vi "MarcusAndMathiasMeetsGoogle.vi"(7 "language":enum16{"de", "en", "sk"}(ring)=enum."en", 8 "error in (no error)":errorcluster, 11 "Input Words":string[](array[string])) -> (0 "error out":errorcluster, 3 "result":string[](array[string]))   [LabVIEW 2015]
uses:
  <vilib>/httpClient/LabVIEWHTTPClient.lvlib
panel:
  in  "Test Value":bool
  out "Numeric":i32
  out "after substring 2":string
  out "json":string
  out "length":i32
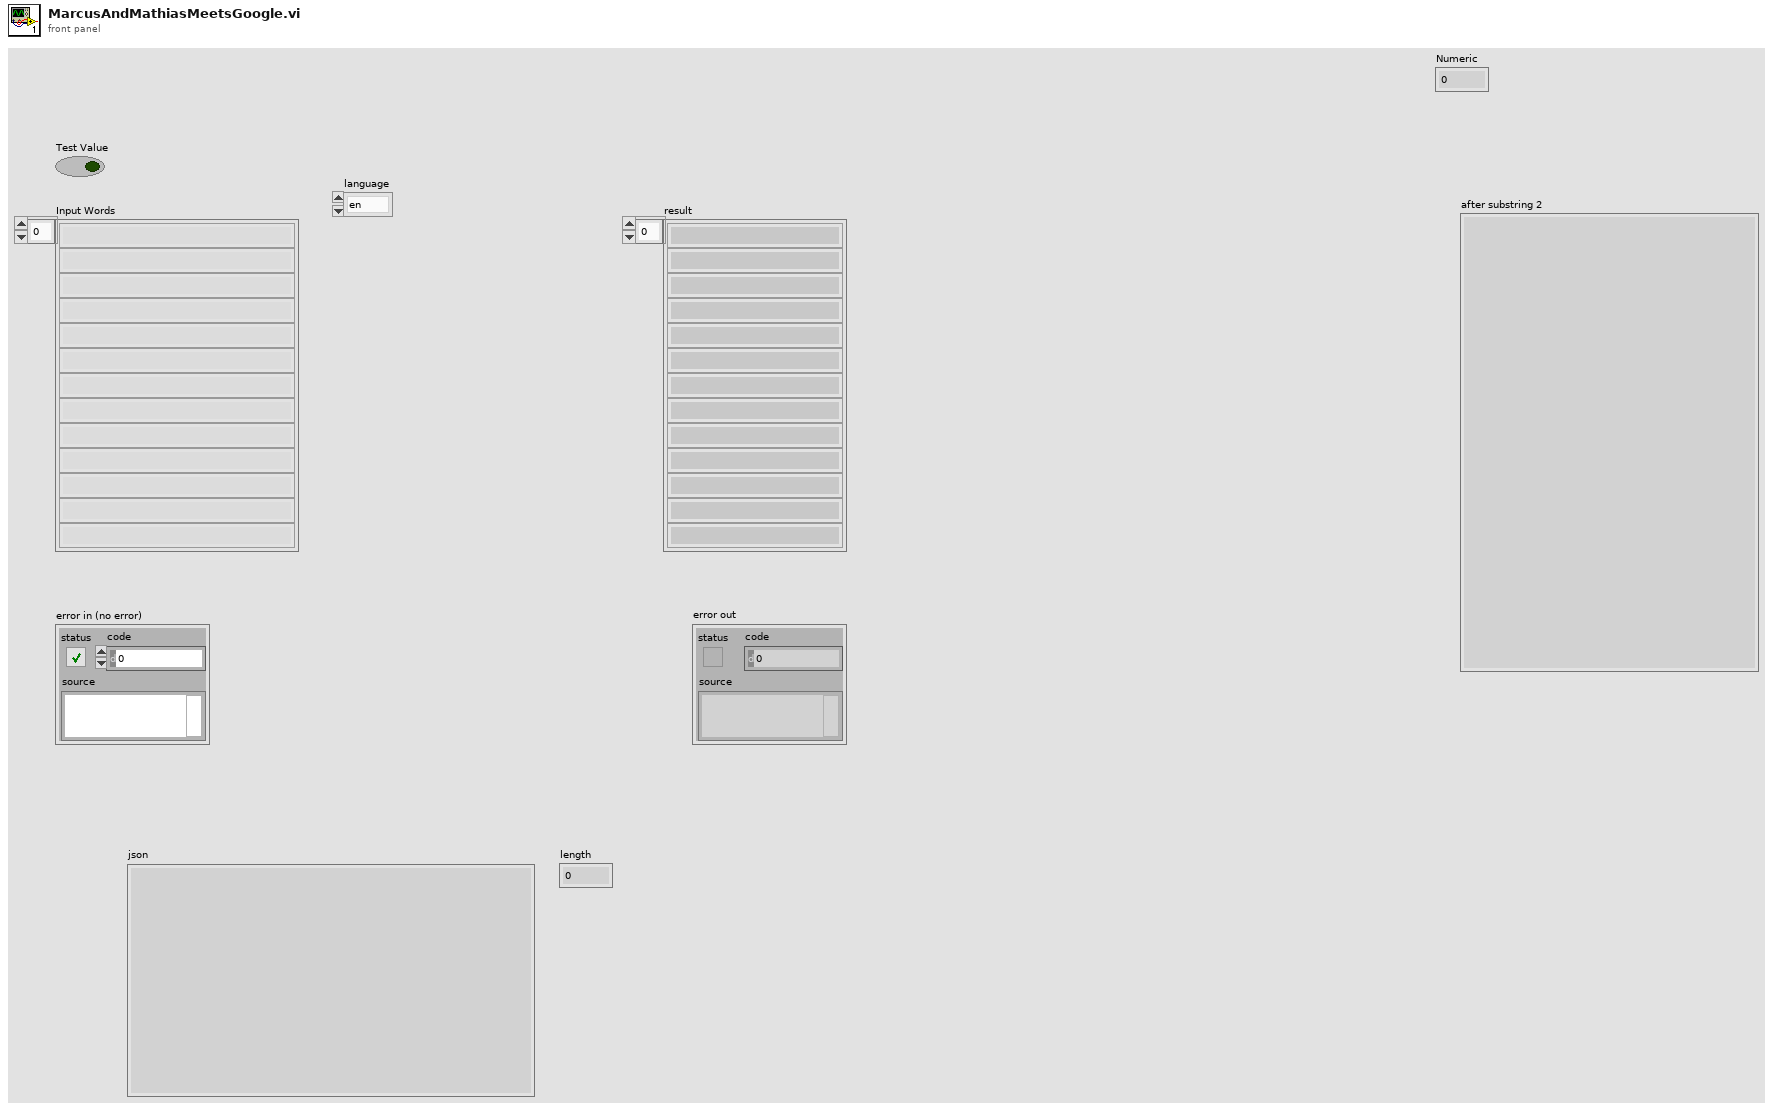
[diagram p1: front panel]
types:
  T1 = typedef "LabVIEWHTTPClient.lvlib/ClientHandle.ctl" = refnum<k1>
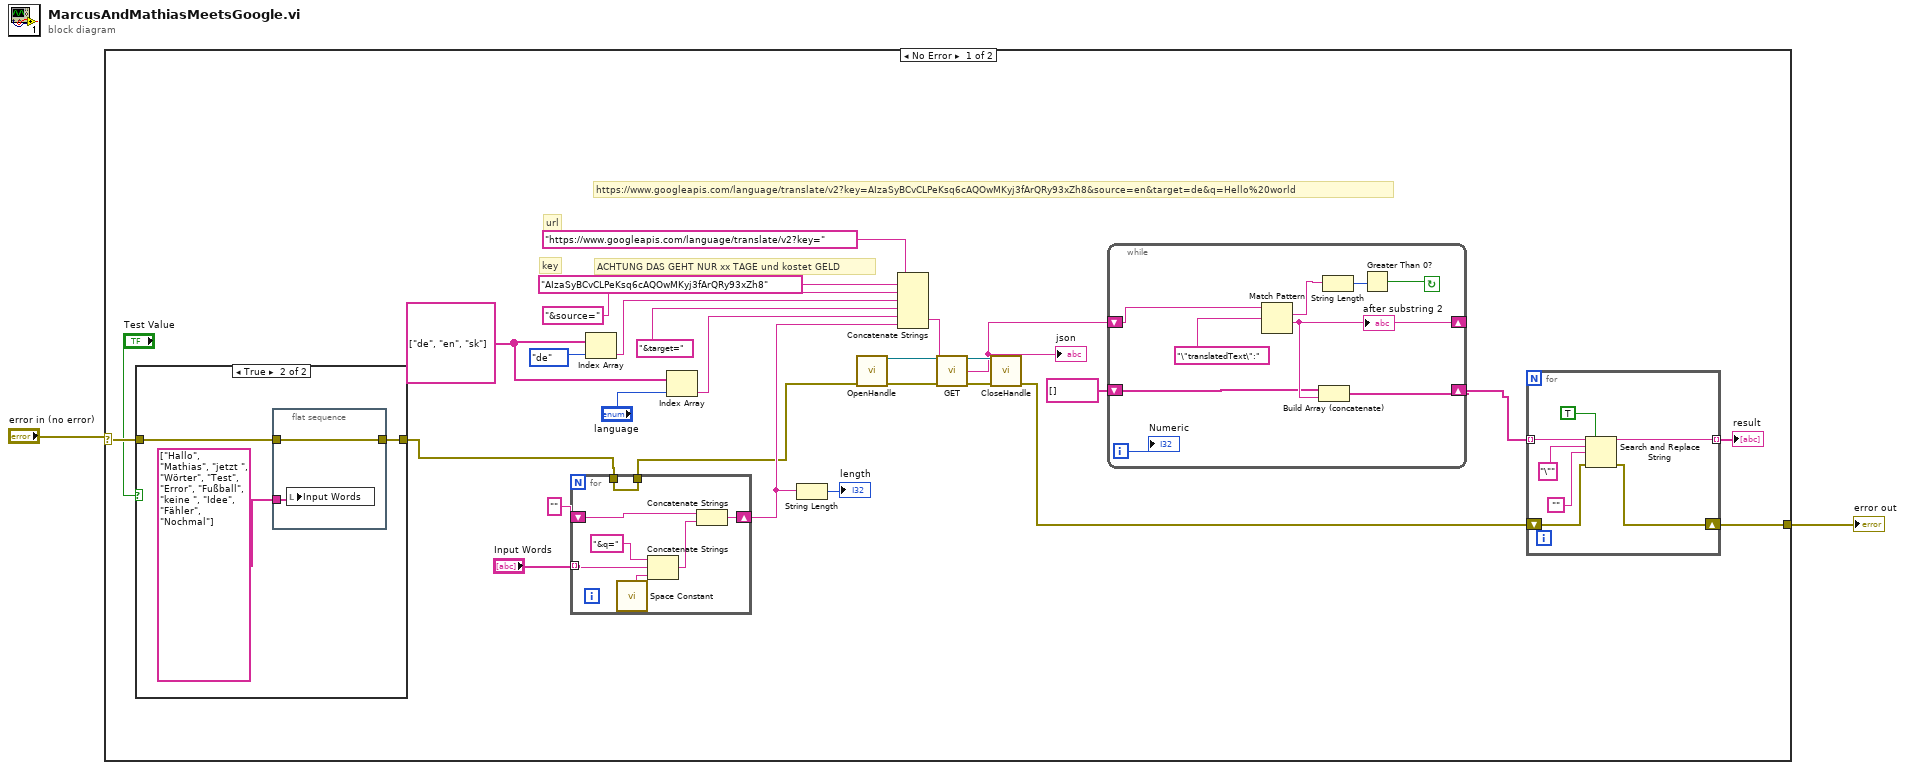
[diagram p0: block diagram]
diagram:
  n1 = case shown="No Error" "error in (no error)" {
    selector: "error in (no error)" -> [w8 w60]
    tunnel: [w7 w60] -> w1
    frame No Error {
      w19 = string[] ["de", "en", "sk"]
      # "ACHTUNG DAS GEHT NUR xx TAGE und kostet GELD"
      # "key"
      # "url"
      # "https://www.googleapis.com/language/translate/v2?key=AIzaSyBCvCLPeKsq6cAQOwMKyj3fArQRy93xZh8&source=en&target=de&q=Hello%20world"
      n2 = case shown="True" "Test Value" {
        tunnel: [w31 w33] -> w5
        tunnel: w8 -> [w31 w32]
        frame False {
        }
        frame True {
          n3 = flat-sequence {
            tunnel: string[] ["Hallo", "Mathias", "jetzt ", "Wörter", "Test", "Error", "Fußball", "keine ", "Idee", "Fähler", "Nochmal"] ("Array 2") -> [w36]
            tunnel: w32 -> [w35]
            tunnel: [w35] -> w33
            frame #0 {
              n4 = local write "Input Words"(w36) -> ()
            }
          }
        }
      }
      n5 = for {
        tunnel: "Input Words" -> [w56] mode=indexing
        shift-right: [w58] -> w9
        shift-left: "" -> [w59]
        tunnel: w5 -> [w53]
        tunnel: [w53] -> w4
        n6 = call <vilib>:"Space Constant.vi"() -> ("String"=w57:string)
        n7 = Concatenate Strings("&q=", w56, w57) -> (w55:string)
        n8 = Concatenate Strings(w59, w55) -> (w58:string)
      }
      n9 = Index Array(array=w19, index=enum16{"de", "en", "sk"}."de") -> (element=w22:string)
      n10 = Index Array(array=w19, index="language") -> (element=w18:string)
      n11 = String Length(string=w9) -> (length=→"length":i32)
      n12 = call <vilib>:"OpenHandle.vi"("error in (no error)"=w4) -> ("client handle out"=w30:T1, "error out"=w29:errorcluster)  [unwired: 13 in]
      n13 = Concatenate Strings("https://www.googleapis.com/language/translate/v2?key=", "AIzaSyBCvCLPeKsq6cAQOwMKyj3fArQRy93xZh8", "&source=", w22, "&target=", w18, w9) -> (w15:string)
      n14 = call <vilib>:"GET.vi"("client handle"=w30, "url"=w15, "error in (no error)"=w29) -> ("client handle out"=w27:T1, "body"=w13:string, "error out"=w28:errorcluster)  [unwired: 9 in, 1 out]
      "json" <- w13
      n15 = call <vilib>:"CloseHandle.vi"("client handle"=w27, "error in (no error)"=w28) -> ("error out"=w10:errorcluster)  [unwired: 13 in]
      n16 = while {
        shift-right: [w45] -> w12
        shift-left: string[] [] -> [w46]
        shift-right: [w47] -> _
        shift-left: w13 -> [w51]
        i -> [w44]
        stop <- w48 continue-if-true
        n17 = Match Pattern(string=w51, regular expression="\"translatedText\":") -> (match substring=w50:string, after substring=w47:string)  [unwired: 1 in, 2 out]
        "after substring 2" <- w47
        n18 = Build Array (concatenate)(w46, w47) -> (w45:string[])
        n19 = String Length(string=w50) -> (length=w49:i32)
        n20 = Greater Than 0?(x=w49) -> (x > 0?=w48:bool)
        "Numeric" <- w44
      }
      n21 = for {
        tunnel: w12 -> [w43] mode=indexing
        tunnel: [w39] -> w11 mode=indexing
        shift-right: [w37] -> w7
        shift-left: w10 -> [w38]
        n22 = Search and Replace String(replace all?=TRUE ("replace all? (F)"), input string=w43, search string="\"", replace string="", error in=w38) -> (result string=w39:string, error out=w37:errorcluster)  [unwired: 3 in, 2 out]
      }
      "result" <- w11
    }
    frame Error {
    }
  }
  "error out" <- w1
